vi "Find Two Peaks (Angle) (SubVI).vi"(8 "Valley or Peak":bool, 11 "Peaks":T1={"Index"=[0, 0, 0], "Angle"=[0.0, 0.0, 0.0]} {"Angle" format="%.14g"}) -> (3 "Index":u16[](array[numeric]))   [LabVIEW 2015]
uses:
  Controls (FPGA)/Peak Index Angle.ctl
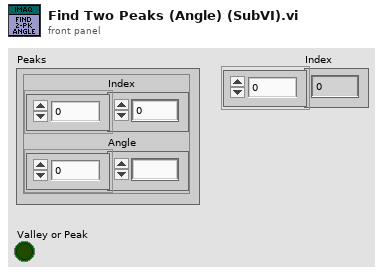
[diagram p1: front panel]
types:
  T1 = typedef "Peak Index Angle.ctl" = cluster{"Index":u16[], "Angle":fxp<+/-,16,3>[]}
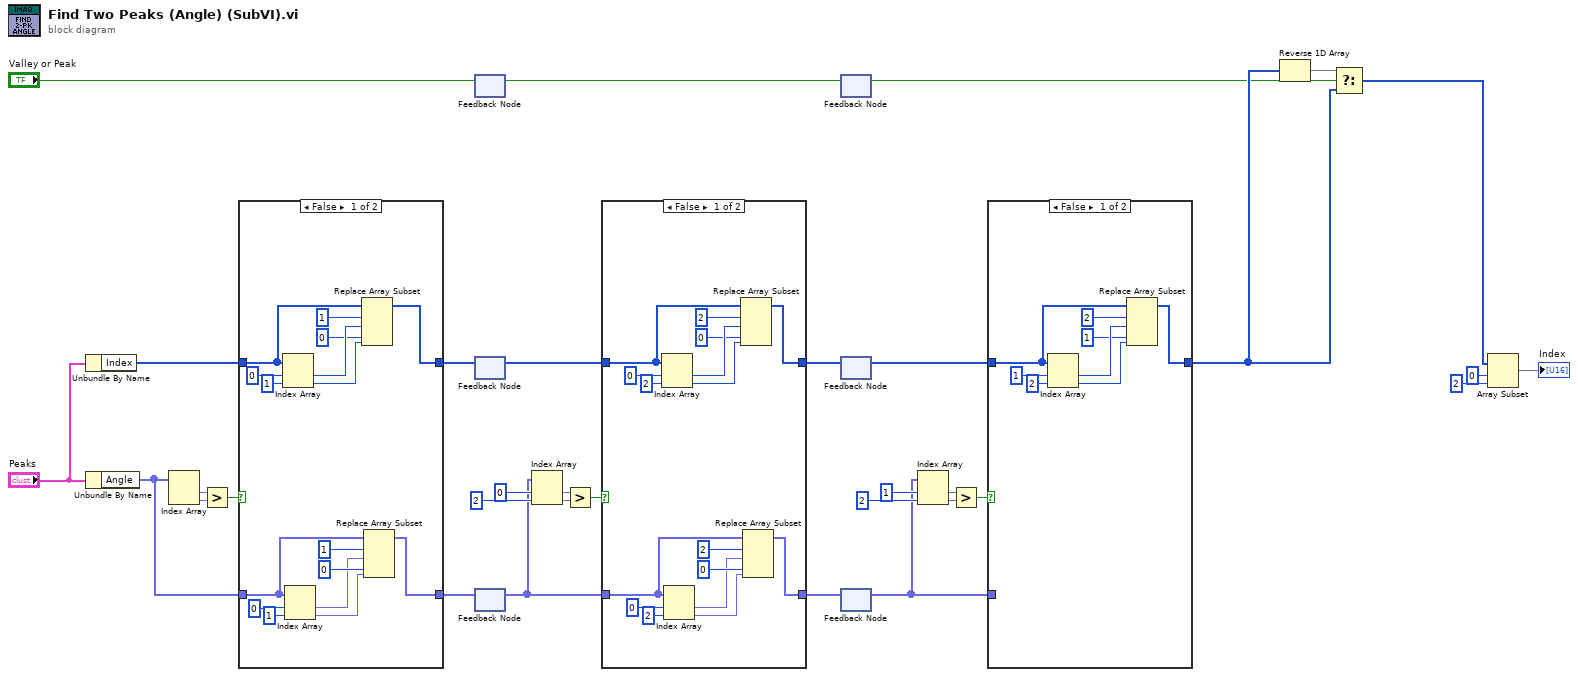
[diagram p0: block diagram]
diagram:
  n1 = Unbundle By Name("Peaks") -> ("Index"=w13:u16[])
  n2 = Unbundle By Name("Peaks") -> ("Angle"=w29:fxp<+/-,16,3>[])
  n3 = Index Array(array=w29) -> (element #1=w31:fxp<+/-,16,3>, element #2=w32:fxp<+/-,16,3>)  [unwired: 2 in]
  n4 = Greater?(x=w31, y=w32) -> (0:w28:bool)
  n5 = case shown="False" w28 {
    tunnel: w29 -> [w49 w51]
    tunnel: [w48 w51] -> w24
    tunnel: w13 -> [w38 w50]
    tunnel: [w39 w50] -> w14
    frame False {
      n6 = Index Array(array=w38, index #1=0 ("index"), index #2=1 ("index")) -> (element #1=w43:u16, element #2=w42:u16)
      n7 = Index Array(array=w49, index #1=0 ("index"), index #2=1 ("index")) -> (element #1=w44:fxp<+/-,16,3>, element #2=w45:fxp<+/-,16,3>)
      n8 = Replace Array Subset(array=w38, new element #1=w43, index #1=1 ("index"), new element #2=w42, index #2=0 ("index")) -> (w39:u16[])
      n9 = Replace Array Subset(array=w49, new element #1=w44, index #1=1 ("index"), new element #2=w45, index #2=0 ("index")) -> (w48:fxp<+/-,16,3>[])
    }
    frame True {
    }
  }
  n10 = feedback-in #1("Valley or Peak") -> ()
  n11 = feedback #1() -> (w1:bool)  [unwired: 1 in]
  n12 = feedback-in #2(w14) -> ()
  n13 = feedback #2() -> (w3:u16[])  [unwired: 1 in]
  n14 = feedback-in #3(w24) -> ()
  n15 = feedback #3() -> (w2:fxp<+/-,16,3>[])  [unwired: 1 in]
  n16 = Index Array(array=w2, index #1=0 ("index"), index #2=2 ("index")) -> (element #1=w26:fxp<+/-,16,3>, element #2=w25:fxp<+/-,16,3>)
  n17 = Greater?(x=w26, y=w25) -> (0:w27:bool)
  n18 = case shown="False" w27 {
    tunnel: w2 -> [w67 w69]
    tunnel: [w66 w69] -> w16
    tunnel: w3 -> [w52 w68]
    tunnel: [w53 w68] -> w15
    frame False {
      n19 = Index Array(array=w52, index #1=0 ("index"), index #2=2 ("index")) -> (element #1=w57:u16, element #2=w56:u16)
      n20 = Index Array(array=w67, index #1=0 ("index"), index #2=2 ("index")) -> (element #1=w62:fxp<+/-,16,3>, element #2=w63:fxp<+/-,16,3>)
      n21 = Replace Array Subset(array=w52, new element #1=w57, index #1=2 ("index"), new element #2=w56, index #2=0 ("index")) -> (w53:u16[])
      n22 = Replace Array Subset(array=w67, new element #1=w62, index #1=2 ("index"), new element #2=w63, index #2=0 ("index")) -> (w66:fxp<+/-,16,3>[])
    }
    frame True {
    }
  }
  n23 = feedback-in #4(w1) -> ()
  n24 = feedback #4() -> (w4:bool)  [unwired: 1 in]
  n25 = feedback-in #5(w15) -> ()
  n26 = feedback #5() -> (w6:u16[])  [unwired: 1 in]
  n27 = feedback-in #6(w16) -> ()
  n28 = feedback #6() -> (w5:fxp<+/-,16,3>[])  [unwired: 1 in]
  n29 = Index Array(array=w5, index #1=1 ("index"), index #2=2 ("index")) -> (element #1=w18:fxp<+/-,16,3>, element #2=w19:fxp<+/-,16,3>)
  n30 = Greater?(x=w18, y=w19) -> (0:w17:bool)
  n31 = case shown="False" w17 {
    tunnel: w5 -> [_ _]
    tunnel: w6 -> [w70 w78]
    tunnel: [w71 w78] -> w8
    frame False {
      n32 = Index Array(array=w70, index #1=1 ("index"), index #2=2 ("index")) -> (element #1=w75:u16, element #2=w74:u16)
      n33 = Replace Array Subset(array=w70, new element #1=w75, index #1=2 ("index"), new element #2=w74, index #2=1 ("index")) -> (w71:u16[])
    }
    frame True {
    }
  }
  n34 = Reverse 1D Array(array=w8) -> (reversed array=w9:u16[])
  n35 = Select(t=w9, s=w4, f=w8) -> (s? t:f=w7:u16[])
  n36 = Array Subset(array=w7, index=0, length=2) -> (→"Index":u16[])
